vi "Write Database.vi"(8 "Error In":errorcluster, 9 "delimiter (\\t)":string=";", 10 "DB Path":path, 11 "Data in":string[][](array[string])) -> (0 "Error Out":errorcluster)   [LabVIEW 2014]
doc: "<B>Copyright</B>: (c) 2015 MHWirth. All rights reserved.\n\nThis subVI writes \"Data in\" in a databse file. Depends on the file extenstion, databse will be Excel or CSV File."
uses:
  <vilib>/addons/_office/excel.llb/Excel Easy Table (str).vi
  <vilib>/Utility/file.llb/Write To Spreadsheet File (string).vi
  <vilib>/Utility/NIReport.llb/NI_report.lvclass
  <vilib>/addons/_office/NI_ReportGenerationToolkit.lvlib
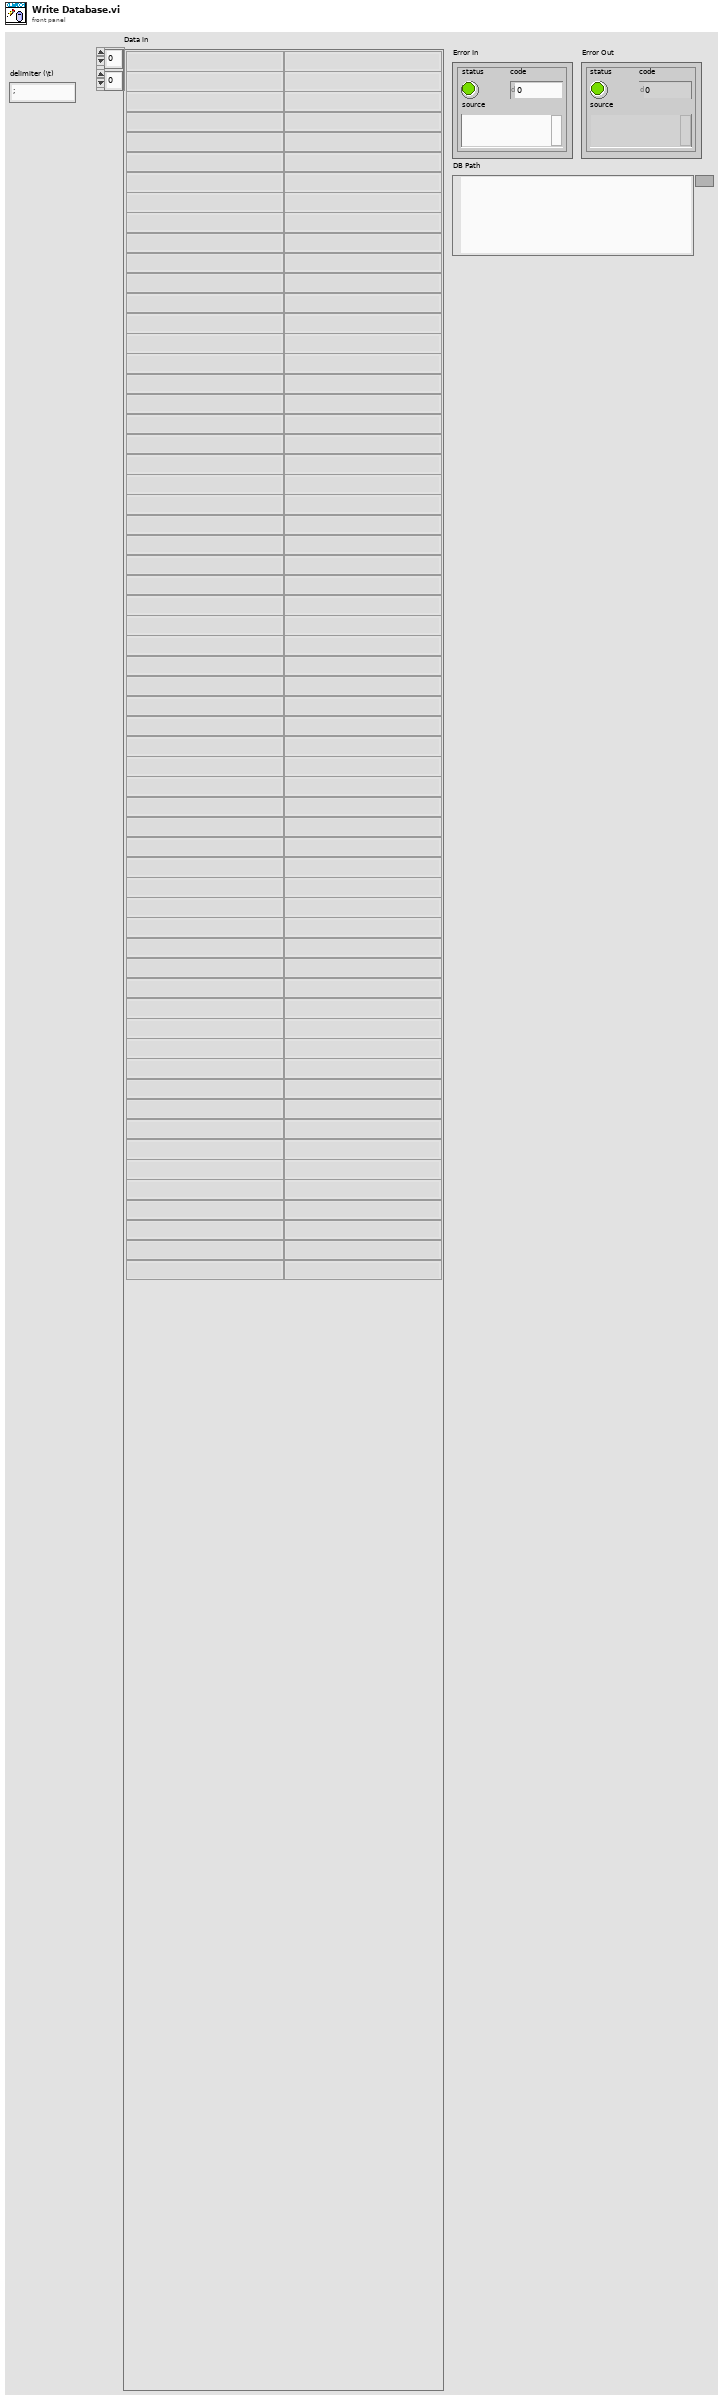
[diagram p1: front panel]
types:
  T1 = enum16{"Standard Report", "HTML", "Word", "Excel"}
  T2 = enum16{"maximized", "minimized", "normal", "no change"}
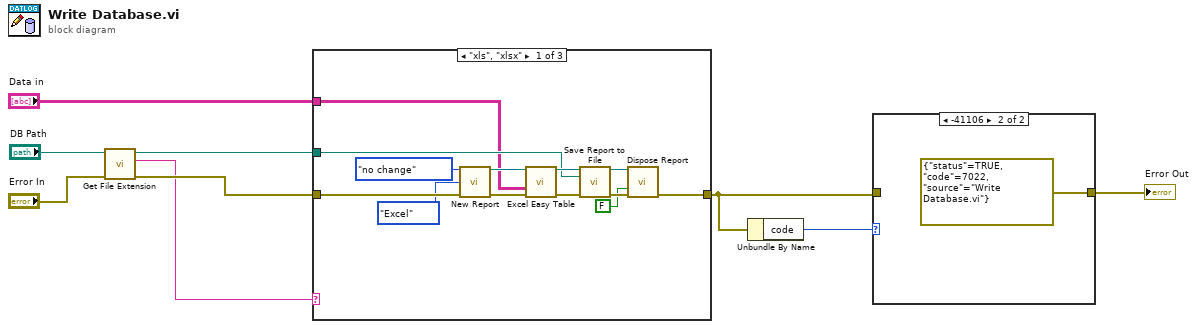
[diagram p0: block diagram]
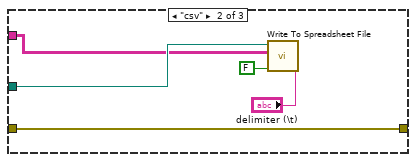
[diagram p3: hidden frame]
diagram:
  n1 = call <vilib>:"Get File Extension.vi"("error in (no error)"="Error In", "file"="DB Path") -> ("error out"=w6:errorcluster, "lowercase file extension"=w4:string, "dup file"=w5:path)  [unwired: 6 in, 1 out]
  n2 = case shown="\"xls\", \"xlsx\"" w4 {
    tunnel: w5 -> [w14 w25 _]
    tunnel: w6 -> [w22 w24 w28]
    tunnel: [w11 w24 w28] -> w2
    tunnel: "Data in" -> [w10 w23 _]
    frame "xls", "xlsx" {
      n3 = call <vilib>:"New Report.vi"("window state (normal)"=T2."no change", "report type"=T1."Excel", "error in (no error)"=w22) -> ("report out"=w18:refnum<class "NI_report.lvclass">, "error out"=w19:errorcluster)  [unwired: 11 in]
      n4 = call-poly <vilib>:"Excel Easy Table.vi"("report in"=w18, "text data"=w10, "error in (no error)"=w19) -> ("report out"=w15:refnum<class "NI_report.lvclass">, "error out"=w17:errorcluster)  [unwired: 8 in, 3 out]
      n5 = call-dynamic "Save Report to File.vi"("report in"=w15, "report file path"=w14, "error in (no error)"=w17) -> ("report out"=w13:refnum<class "NI_report.lvclass">, "error out"=w16:errorcluster)  [unwired: 11 in]
      n6 = call-dynamic "Dispose Report.vi"("report in"=w13, "save changes? (F)"=FALSE, "error in (no error)"=w16) -> ("error out"=w11:errorcluster)  [unwired: 12 in]
    }
    frame "csv" {
      n7 = call-poly <vilib>:"Write To Spreadsheet File.vi"("delimiter (\\t)"="delimiter (\\t)", "append to file? (new file:F)"=FALSE, "2D data"=w23, "file path (dialog if empty)"=w25) -> ()  [unwired: 4 in, 1 out]
    }
    frame "unknown", Default {
    }
  }
  n8 = Unbundle By Name(w2) -> ("code"=w1:i32)
  n9 = case shown="-41106" w1 {
    tunnel: [w29 errorcluster {"status"=TRUE, "code"=7022, "source"="Write Database.vi"} ("error out")] -> w3
    tunnel: w2 -> [w29 _]
    frame 0, Default {
    }
    frame -41106 {
    }
  }
  "Error Out" <- w3
